vi "PH_Interaction.get running at - Information.vi"(1 "Instance":string) -> (0 "Running @ - Information":string)   [LabVIEW 2014, in "PH_Common.lvlib"]
uses:
  PH_Common.lvlib
  CS_Core/CSSystem/CSSystemLib/CSSystemLib.lvlib
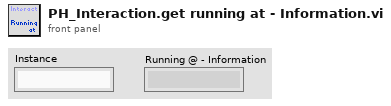
[diagram p1: front panel]
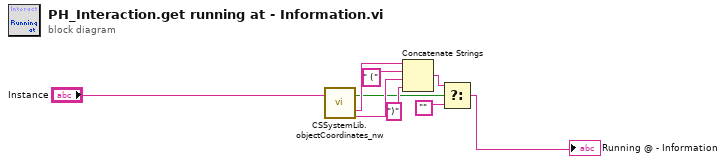
[diagram p0: block diagram]
diagram:
  n1 = call "CSSystemLib.objectCoordinates_nw.vi"("name"="Instance") -> ("obj exists"=w1:bool, "systemID"=w4:string, "node"=w7:string)  [unwired: 15 in, 1 out]
  n2 = Concatenate Strings(w4, " (" ("string"), w7, ")" ("string")) -> (w5:string)
  n3 = Select(t=w5, s=w1, f="") -> (s? t:f=→"Running @ - Information":string)
